vi "_fgv_rep_caps.vi"(5 "RepCapName in (\"\")":string, 6 "Repeated Capabilities (empty)":T1[](array[typedef]), 7 "Operation":T2=enum."Get Cmd Value", 8 "error in":errorcluster caption="error in (no error)", 9 "RepCapNameCmdValue in (\"\")":string, 10 "RepCapNameID in (\"\")":string, 11 "VISA resource name":refnum<visa-resource-name>) -> (0 "error out":errorcluster, 1 "RepCap count out":i32, 2 "CmdValue out":string, 3 "VISA resource name out":refnum<visa-resource-name>)   [LabVIEW 2020, in "Rohde&Schwarz RTx Oscilloscopes.lvlib" / "rsidr_core.lvlib"]
uses:
  rsidr_core.lvlib
  _type_Operation_Fgv_RepCap.ctl
  type_Input_Format_RepCap.ctl
  type_Error_Codes.ctl
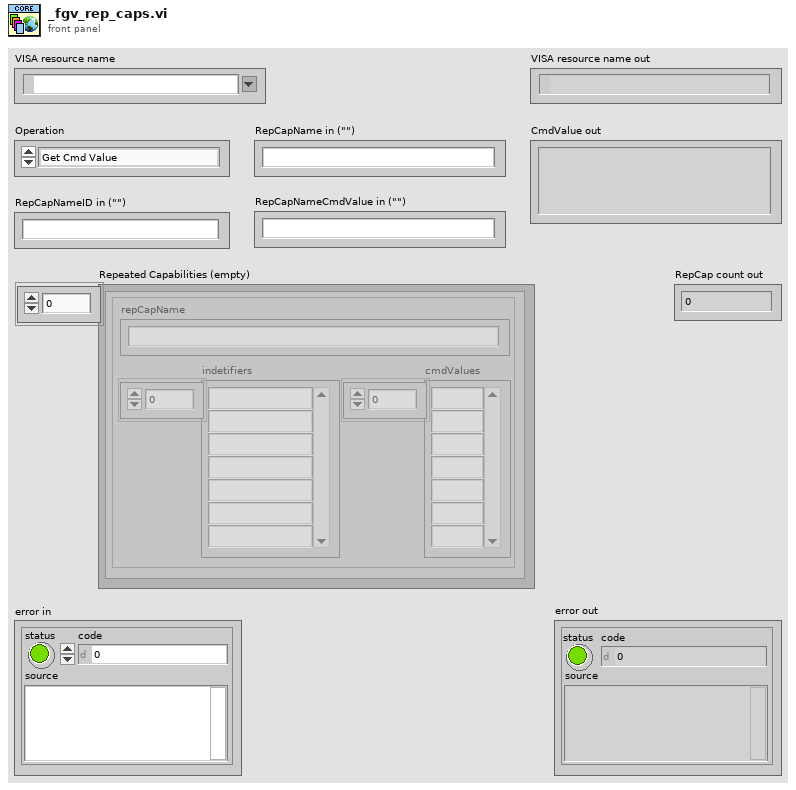
[diagram p1: front panel]
types:
  T1 = typedef "Rohde&Schwarz RTx Oscilloscopes.lvlib/rsidr_core.lvlib/type_Input_Format_RepCap.ctl" = cluster{"repCapName":string, "indetifiers":string[], "cmdValues":string[]}
  T2 = typedef "Rohde&Schwarz RTx Oscilloscopes.lvlib/rsidr_core.lvlib/_type_Operation_Fgv_RepCap.ctl" = enum16{"Initialize", "Get Cmd Value", "Reset Rep Cap", "Add Rep Cap", "Remove Rep Cap", "Get Rep Cap ID range", "Get Count", "Clear", "Find Name from NameID", "Get First NameID"}
  T3 = typedef "Rohde&Schwarz RTx Oscilloscopes.lvlib/rsidr_core.lvlib/type_Error_Codes.ctl" = enum16{"No_error", "VISA_err_ResourceNotFound", "VISA_err_Timeout", "VISA_warn_MoreDataAvailable", "RS_err_MissingCallback", "RS_err_InvalidAttribute", "RS_err_InvalidValue", "RS_err_UnknownResource", "RS_err_AlreadyInitialized", "RS_err_InstrumentStatus", "RS_err_BadRepCapName", "RS_err_TypesMismatch", "RS_err_ValueNotSupported", "RS_err_InvalidRngTable", "RS_err_IDqueryFail", "RS_err_UnexpResponse", "VISA_warn_ConfigNotLoaded", "RS_err_AttributeNotReadable", "RS_err_AttributeNotWritable", "RS_err_InstrumentType", "RS_err_InstrumentOption", "VISA_err_InvalidSize", "RS_err_ReliabilityIndicator", "VISA_warn_UnknownStatus", "VISA_warn_TermCharRead", "VISA_err_IO_error", "RS_err_FunctionNotSupported", "VISA_warn_QueueEmpty"}
  T4 = typedef "Rohde&Schwarz RTx Oscilloscopes.lvlib/rsidr_core.lvlib/_type_RepCap_Type.ctl" = enum16{"Arbitrary", "SequentialNull", "Sequential"}
  T5 = cluster{"repCapName":string, "RepCap Type out":T4, "RepCap IDs out":variant}
  T6 = cluster{"repCapName":string, "RepCap Type out":T4, "RepCap IDs out":variant}[]
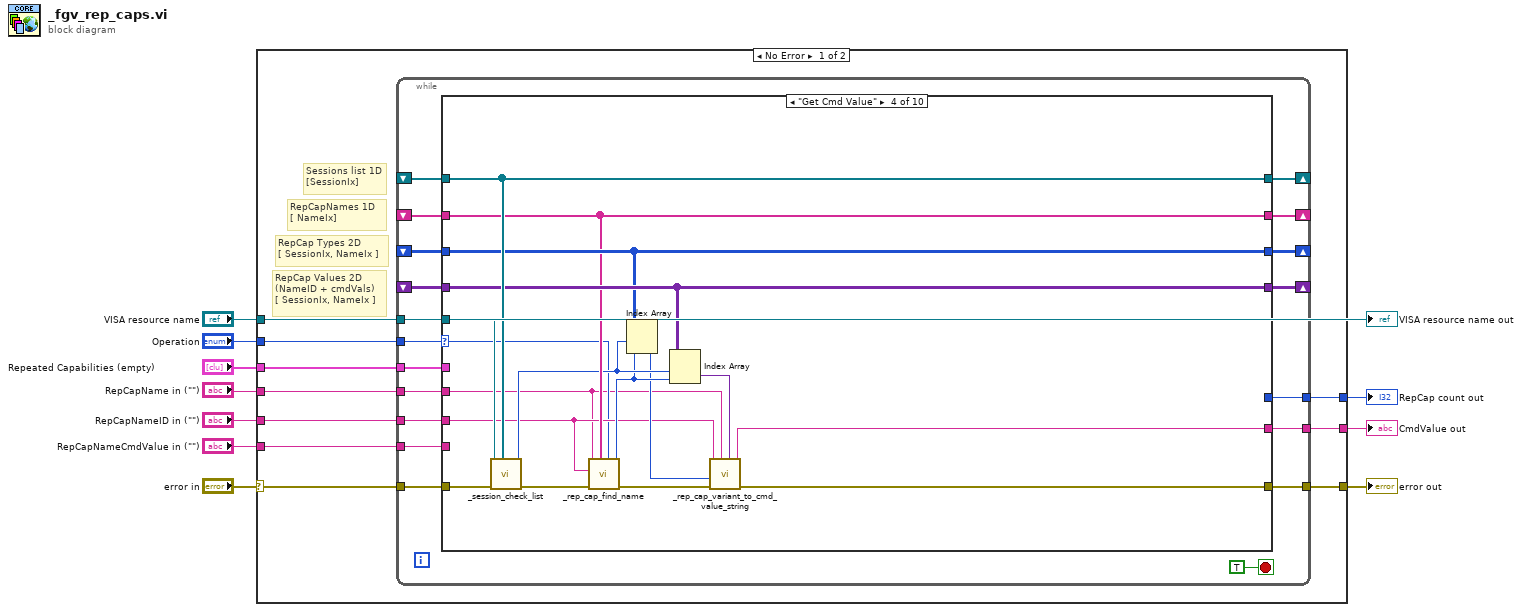
[diagram p0: block diagram]
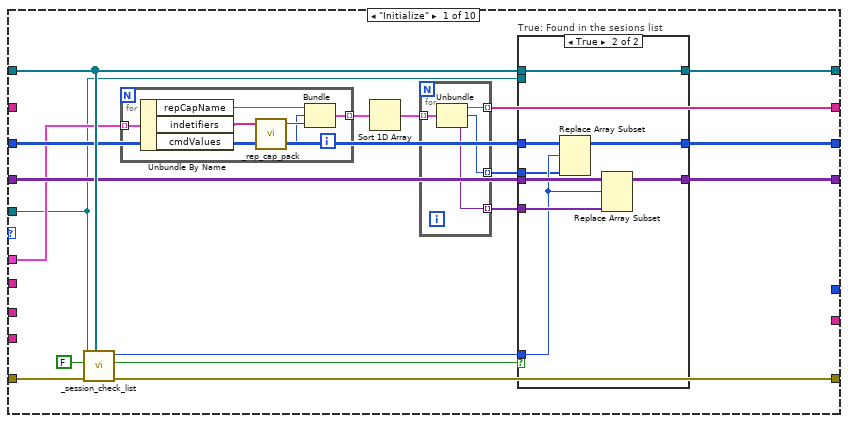
[diagram p2: hidden frame]
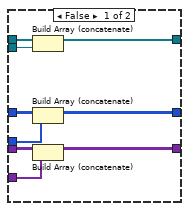
[diagram p3: hidden frame]
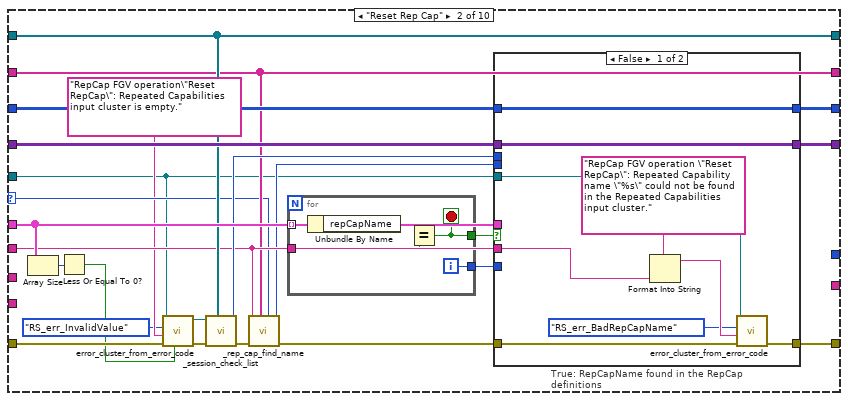
[diagram p4: hidden frame]
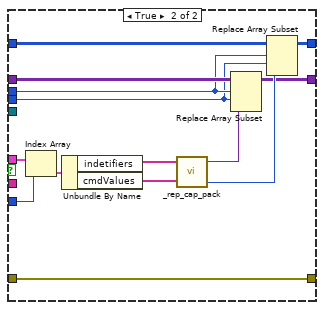
[diagram p5: hidden frame]
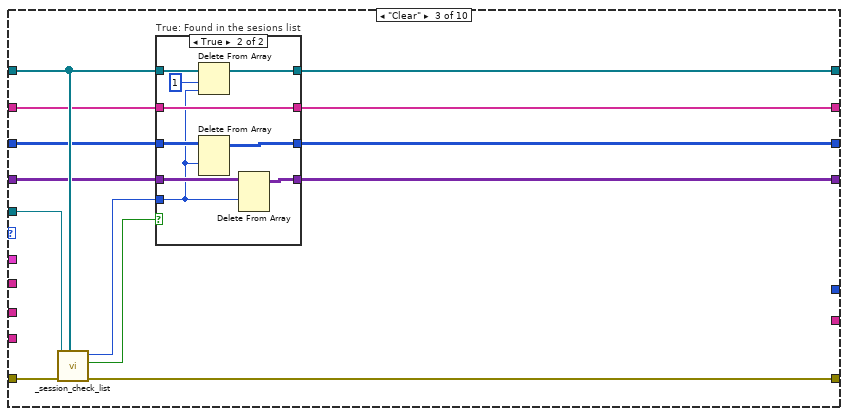
[diagram p6: hidden frame]
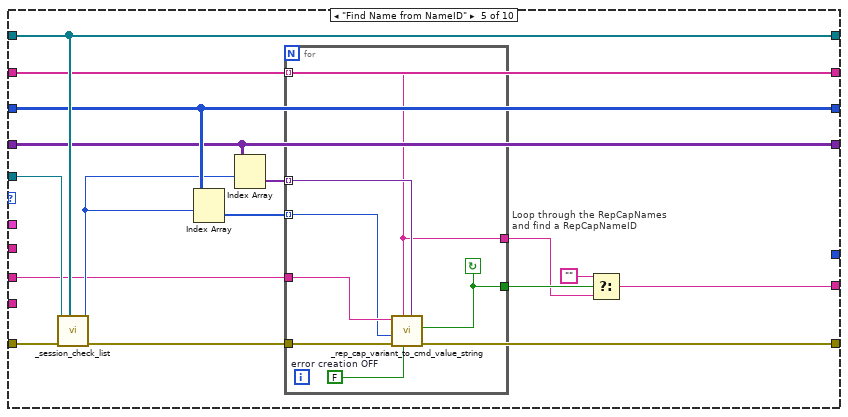
[diagram p8: hidden frame]
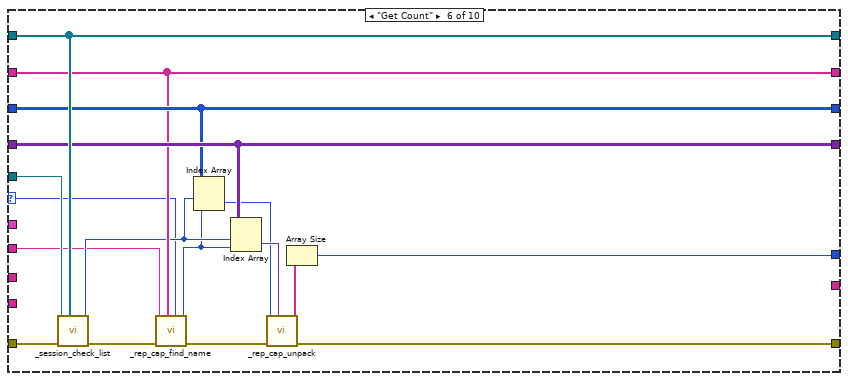
[diagram p9: hidden frame]
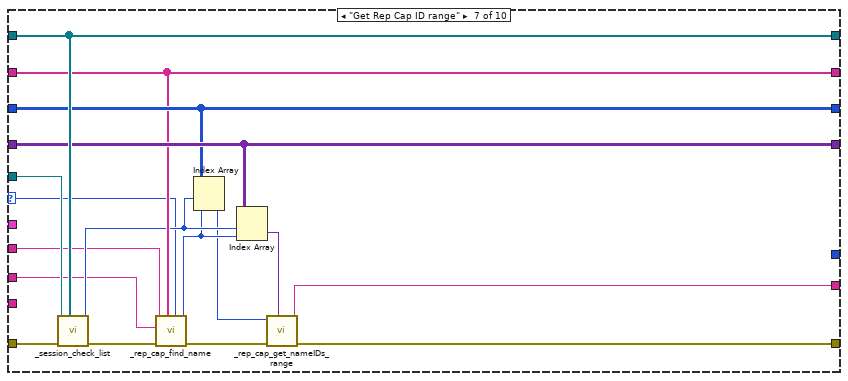
[diagram p10: hidden frame]
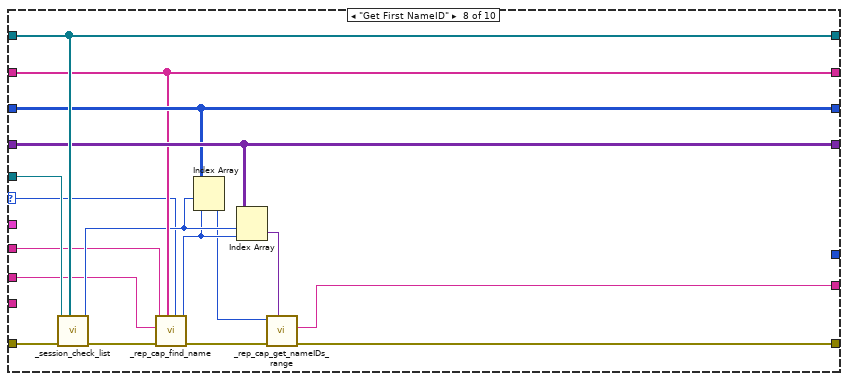
[diagram p11: hidden frame]
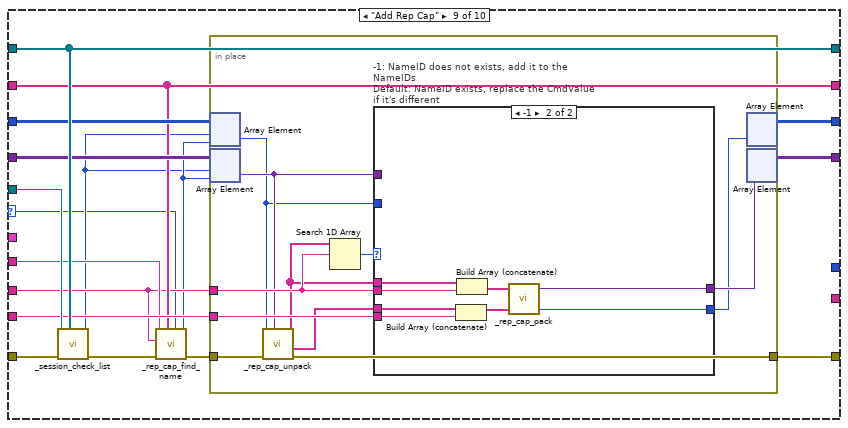
[diagram p12: hidden frame]
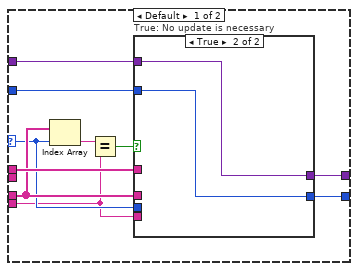
[diagram p13: hidden frame]
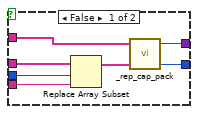
[diagram p14: hidden frame]
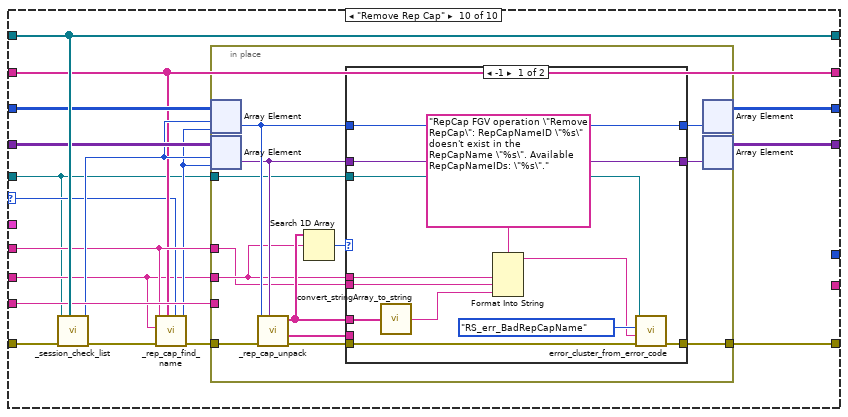
[diagram p15: hidden frame]
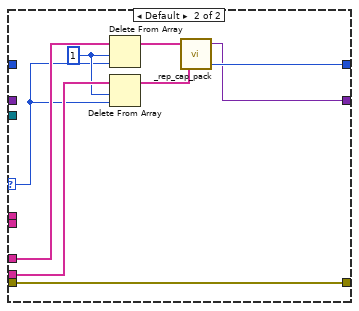
[diagram p16: hidden frame]
diagram:
  n1 = case shown="No Error" "error in" {
    selector: "error in" -> [w12 w360]
    tunnel: "Operation" -> [w20 _]
    tunnel: "VISA resource name" -> [w19 _]
    tunnel: [w13 w360] -> w9
    tunnel: "Repeated Capabilities (empty)" -> [w18 _]
    tunnel: "RepCapName in (\"\")" -> [w17 _]
    tunnel: "RepCapNameID in (\"\")" -> [w16 _]
    tunnel: [w15 _] -> w4
    tunnel: "RepCapNameCmdValue in (\"\")" -> [w14 _]
    tunnel: [w11 _] -> w1
    frame No Error {
      # "RepCap Values 2D\n(NameID + cmdVals)\n[ SessionIx, NameIx ]"
      # "Sessions list 1D\n[SessionIx]"
      # "RepCapNames 1D\n[ NameIx]"
      # "RepCap Types 2D\n[ SessionIx, NameIx ]"
      n2 = while {
        tunnel: w20 -> [w26]
        tunnel: [w39] -> w13
        tunnel: w19 -> [w23]
        tunnel: w18 -> [w37]
        tunnel: w17 -> [w36]
        tunnel: w16 -> [w35]
        tunnel: [w34] -> w15
        tunnel: w14 -> [w33]
        tunnel: w12 -> [w24]
        shift-right: [w31] -> _
        shift-left: _ -> [w32]
        shift-right: [w27] -> _
        shift-left: _ -> [w30]
        shift-right: [w28] -> _
        shift-left: _ -> [w29]
        shift-right: [w22] -> _
        shift-left: _ -> [w25]
        tunnel: [w21] -> w11
        stop <- TRUE stop-if-true
        n3 = case shown="\"Get Cmd Value\"" w26 {
          selector: w26 -> [_ w91 _ w165 _ w210 w227 w244 w254 w311]
          tunnel: [w56 w107 w149 w180 w185 w206 w222 w239 w270 w325] -> w39
          tunnel: w23 -> [w40 w86 w140 w177 w194 w218 w235 w252 w268 w309]
          tunnel: w37 -> [w43 w104 _ _ _ _ _ _ _ _]
          tunnel: w36 -> [_ w97 _ w164 _ w209 w226 w243 w259 w315]
          tunnel: w35 -> [_ _ _ w166 w187 _ w220 w238 w257 w310]
          tunnel: [_ _ _ w179 w182 _ w221 w237 _ _] -> w34
          tunnel: w33 -> [_ _ _ _ _ _ _ _ w262 w318]
          tunnel: w24 -> [w41 w109 w150 w178 w195 w219 w236 w253 w269 w324]
          tunnel: w32 -> [w48 w106 w141 w175 w190 w216 w233 w250 w266 w322]
          tunnel: [w45 w102 w138 w175 w190 w216 w233 w250 w263 w319] -> w31
          tunnel: w30 -> [_ w96 w145 w171 w191 w213 w230 w247 w258 w314]
          tunnel: w29 -> [w51 w105 w143 w174 w192 w215 w232 w249 w265 w321]
          tunnel: [w46 w103 w139 w174 w192 w215 w232 w249 w264 w320] -> w28
          tunnel: [w42 w96 w144 w171 w191 w213 w230 w247 w258 w314] -> w27
          tunnel: w25 -> [w53 w100 w147 w176 w193 w217 w234 w251 w267 w323]
          tunnel: [w52 w100 w146 w176 w193 w217 w234 w251 w267 w323] -> w22
          tunnel: [_ _ _ _ _ w204 _ _ _ _] -> w21
          frame "Initialize" {
            n4 = call "_session_check_list.vi"("VISA resource names in"=w53, "error in"=w41, "Error if not found (T)"=FALSE, "VISA resource name"=w40) -> ("error out"=w56:errorcluster, "Found in the list"=w54:bool, "Session list index out"=w50:i32)  [unwired: 5 in]
            n5 = for {
              tunnel: w43 -> [w85] mode=indexing
              tunnel: [w84] -> w55 mode=indexing
              n6 = Unbundle By Name(w85) -> ("repCapName"=w81:string, "indetifiers"=w83:string[], "cmdValues"=w79:string[])
              n7 = call "_rep_cap_pack.vi"("RepCapName CmdValues"=w79, "RepCapName IDs"=w83) -> ("RepCap Type out"=w80:T4, "RepCap IDs out"=w82:variant)  [unwired: 2 in]
              n8 = Bundle("repCapName"=w81, "RepCap Type out"=w80, "RepCap IDs out"=w82) -> (w84:T5)  [unwired: 1 in]
            }
            n9 = Sort 1D Array(array=w55) -> (sorted array=w57:T6)
            n10 = for {
              tunnel: w57 -> [w78] mode=indexing
              tunnel: [w76] -> w42 mode=indexing
              tunnel: [w77] -> w47 mode=indexing
              tunnel: [w75] -> w49 mode=indexing
              n11 = Unbundle(w78) -> ("repCapName"=w76:string, "RepCap Type out"=w77:T4, "RepCap IDs out"=w75:variant)
            }
            n12 = case "True: Found in the sesions list" shown="True" w54 {
              tunnel: w53 -> [w66 w74]
              tunnel: [w65 w74] -> w52
              tunnel: w51 -> [w63 w73]
              tunnel: w50 -> [_ w68]
              tunnel: w49 -> [w58 w71]
              tunnel: w48 -> [w61 w72]
              tunnel: w47 -> [w59 w67]
              tunnel: w40 -> [w64 _]
              tunnel: [w62 w70] -> w46
              tunnel: [w60 w69] -> w45
              frame False {
                n13 = Build Array (concatenate)(w66, w64) -> (w65:refnum<visa-resource-name>[])
                n14 = Build Array (concatenate)(w63, w59) -> (w62:T4[][])
                n15 = Build Array (concatenate)(w61, w58) -> (w60:variant[][])
              }
              frame True {
                n16 = Replace Array Subset(array=w73, new element=w67, index (row)=w68) -> (w70:T4[][])  [unwired: 1 in]
                n17 = Replace Array Subset(array=w72, new element=w71, index (row)=w68) -> (w69:variant[][])  [unwired: 1 in]
              }
            }
          }
          frame "Reset Rep Cap" {
            n18 = Array Size(array=w104) -> (size(s)=w108:i32)
            n19 = Less Or Equal To 0?(x=w108) -> (x <= 0?=w87:bool)
            n20 = call "error_cluster_from_error_code.vi"("Error Creation Enabled (True)"=w87, "error in"=w109, "Error Message (\"\")"="RepCap FGV operation\"Reset RepCap\": Repeated Capabilities input cluster is empty." ("format string"), "Error Enum in"=type_Error_Codes."RS_err_InvalidValue", "VISA resource name"=w86) -> ("error out"=w101:errorcluster, "VISA resource name out"=w90:refnum<visa-resource-name>)  [unwired: 5 in]
            n21 = call "_session_check_list.vi"("VISA resource names in"=w100, "error in"=w101, "VISA resource name"=w90) -> ("error out"=w98:errorcluster, "Session list index out"=w99:i32)  [unwired: 6 in, 1 out]
            n22 = call "_rep_cap_find_name.vi"("Operation for error msg"=w91, "RepCapNames in"=w96, "error in"=w98, "RepCapName to search"=w97) -> ("error out"=w94:errorcluster, "Index out"=w95:i32)  [unwired: 6 in]
            n23 = for {
              tunnel: w104 -> [w137] mode=indexing
              tunnel: w97 -> [w134]
              tunnel: [w133] -> w93
              tunnel: [w135] -> w92
              i -> [w135]
              stop <- w133 stop-if-true
              n24 = Unbundle By Name(w137) -> ("repCapName"=w136:string)
              n25 = Equal?(x=w136, y=w134) -> (x = y?=w133:bool)
            }
            n26 = case "True: RepCapName found in the RepCap definitions" shown="False" w93 {
              tunnel: w94 -> [w116 w119]
              tunnel: w104 -> [_ w131]
              tunnel: w92 -> [_ w132]
              tunnel: w105 -> [w118 w126]
              tunnel: w106 -> [w117 w123]
              tunnel: [w118 w127] -> w103
              tunnel: [w117 w124] -> w102
              tunnel: w99 -> [_ w122]
              tunnel: w95 -> [_ w121]
              tunnel: [w115 w119] -> w107
              tunnel: w97 -> [w113 _]
              tunnel: w86 -> [w112 _]
              frame False {
                n27 = Format Into String(format string="RepCap FGV operation \"Reset RepCap\": Repeated Capability name \"%s\" could not be found in the Repeated Capabilities input cluster.", w113) -> (resulting string=w111:string)  [unwired: 2 in, 1 out]
                n28 = call "error_cluster_from_error_code.vi"("error in"=w116, "Error Message (\"\")"=w111, "Error Enum in"=type_Error_Codes."RS_err_BadRepCapName", "VISA resource name"=w112) -> ("error out"=w115:errorcluster)  [unwired: 6 in, 1 out]
              }
              frame True {
                n29 = Index Array(array=w131, index=w132) -> (element=w130:T1)
                n30 = Unbundle By Name(w130) -> ("indetifiers"=w129:string[], "cmdValues"=w128:string[])
                n31 = call "_rep_cap_pack.vi"("RepCapName CmdValues"=w128, "RepCapName IDs"=w129) -> ("RepCap Type out"=w125:T4, "RepCap IDs out"=w120:variant)  [unwired: 2 in]
                n32 = Replace Array Subset(array=w123, new element=w120, index (row)=w122, index (col)=w121) -> (w124:variant[][])
                n33 = Replace Array Subset(array=w126, new element=w125, index (row)=w122, index (col)=w121) -> (w127:T4[][])
              }
            }
          }
          frame "Clear" {
            n34 = call "_session_check_list.vi"("VISA resource names in"=w147, "error in"=w150, "VISA resource name"=w140) -> ("error out"=w149:errorcluster, "Found in the list"=w148:bool, "Session list index out"=w142:i32)  [unwired: 6 in]
            n35 = case "True: Found in the sesions list" shown="True" w148 {
              tunnel: w147 -> [w154 w158]
              tunnel: [w154 w157] -> w146
              tunnel: w145 -> [w153 w159]
              tunnel: [w153 w159] -> w144
              tunnel: w143 -> [w152 w163]
              tunnel: w142 -> [_ w156]
              tunnel: w141 -> [w151 w162]
              tunnel: [w152 w161] -> w139
              tunnel: [w151 w160] -> w138
              frame False {
              }
              frame True {
                n36 = Delete From Array(array=w158, length=1, index=w156) -> (array with subset deleted=w157:refnum<visa-resource-name>[])  [unwired: 1 out]
                n37 = Delete From Array(array=w163, index (row)=w156) -> (array with subset deleted=w161:T4[][])  [unwired: 2 in, 1 out]
                n38 = Delete From Array(array=w162, index (row)=w156) -> (array with subset deleted=w160:variant[][])  [unwired: 2 in, 1 out]
              }
            }
          }
          frame "Get Cmd Value" {
            n39 = call "_session_check_list.vi"("VISA resource names in"=w176, "error in"=w178, "VISA resource name"=w177) -> ("error out"=w173:errorcluster, "Session list index out"=w170:i32)  [unwired: 6 in, 1 out]
            n40 = call "_rep_cap_find_name.vi"("Operation for error msg"=w165, "RepCapNames in"=w171, "error in"=w173, "RepCapNameID for error msg (\"\")"=w166, "RepCapName to search"=w164) -> ("error out"=w172:errorcluster, "Index out"=w169:i32)  [unwired: 5 in]
            n41 = Index Array(array=w174, index (row)=w170, index (col)=w169) -> (element=w168:T4)
            n42 = Index Array(array=w175, index (row)=w170, index (col)=w169) -> (element=w167:variant)
            n43 = call "_rep_cap_variant_to_cmd_value_string.vi"("RepCap value in"=w167, "RepCapName in"=w164, "error in"=w172, "RepCap Type in"=w168, "RepCapName ID in"=w166) -> ("error out"=w180:errorcluster, "CmdValue out"=w179:string)  [unwired: 4 in, 1 out]
          }
          frame "Find Name from NameID" {
            n44 = call "_session_check_list.vi"("VISA resource names in"=w193, "error in"=w195, "VISA resource name"=w194) -> ("error out"=w185:errorcluster, "Session list index out"=w189:i32)  [unwired: 6 in, 1 out]
            n45 = Index Array(array=w192, index (row)=w189) -> (element=w186:T4[])  [unwired: 1 in]
            n46 = Index Array(array=w190, index (row)=w189) -> (element=w188:variant[])  [unwired: 1 in]
            n47 = for "Loop through the RepCapNames\nand find a RepCapNameID" {
              tunnel: w191 -> [w198] mode=indexing
              tunnel: w188 -> [w201] mode=indexing
              tunnel: w187 -> [w202]
              tunnel: w186 -> [w200] mode=indexing
              tunnel: w185 -> [w199]
              tunnel: [w197] -> w184
              tunnel: [w198] -> w183
              stop <- w197 continue-if-true
              w196 = FALSE  # error creation OFF
              n48 = call "_rep_cap_variant_to_cmd_value_string.vi"("RepCap value in"=w201, "Error creation enabled (T)"=w196, "RepCapName in"=w198, "error in"=w199, "RepCap Type in"=w200, "RepCapName ID in"=w202) -> ("Error occured"=w197:bool)  [unwired: 3 in, 2 out]
            }
            n49 = Select(t="" ("Empty String Constant"), s=w184, f=w183) -> (s? t:f=w182:string)
          }
          frame "Get Count" {
            n50 = call "_session_check_list.vi"("VISA resource names in"=w217, "error in"=w219, "VISA resource name"=w218) -> ("error out"=w214:errorcluster, "Session list index out"=w212:i32)  [unwired: 6 in, 1 out]
            n51 = call "_rep_cap_find_name.vi"("Operation for error msg"=w210, "RepCapNames in"=w213, "error in"=w214, "RepCapName to search"=w209) -> ("error out"=w207:errorcluster, "Index out"=w211:i32)  [unwired: 6 in]
            n52 = Index Array(array=w215, index (row)=w212, index (col)=w211) -> (element=w203:T4)
            n53 = Index Array(array=w216, index (row)=w212, index (col)=w211) -> (element=w208:variant)
            n54 = call "_rep_cap_unpack.vi"("RepCap Value in"=w208, "error in"=w207, "RepCap Type in"=w203) -> ("error out"=w206:errorcluster, "RepCapName IDs"=w205:string[])  [unwired: 6 in, 1 out]
            n55 = Array Size(array=w205) -> (size(s)=w204:i32)
          }
          frame "Get Rep Cap ID range" {
            n56 = call "_session_check_list.vi"("VISA resource names in"=w234, "error in"=w236, "VISA resource name"=w235) -> ("error out"=w231:errorcluster, "Session list index out"=w229:i32)  [unwired: 6 in, 1 out]
            n57 = call "_rep_cap_find_name.vi"("Operation for error msg"=w227, "RepCapNames in"=w230, "error in"=w231, "RepCapNameID for error msg (\"\")"=w220, "RepCapName to search"=w226) -> ("error out"=w225:errorcluster, "Index out"=w228:i32)  [unwired: 5 in]
            n58 = Index Array(array=w232, index (row)=w229, index (col)=w228) -> (element=w224:T4)
            n59 = Index Array(array=w233, index (row)=w229, index (col)=w228) -> (element=w223:variant)
            n60 = call "_rep_cap_get_nameIDs_range.vi"("RepCap value in"=w223, "error in"=w225, "RepCap Type in"=w224) -> ("error out"=w222:errorcluster, "ID range out"=w221:string)  [unwired: 6 in, 1 out]
          }
          frame "Get First NameID" {
            n61 = call "_session_check_list.vi"("VISA resource names in"=w251, "error in"=w253, "VISA resource name"=w252) -> ("error out"=w248:errorcluster, "Session list index out"=w246:i32)  [unwired: 6 in, 1 out]
            n62 = call "_rep_cap_find_name.vi"("Operation for error msg"=w244, "RepCapNames in"=w247, "error in"=w248, "RepCapNameID for error msg (\"\")"=w238, "RepCapName to search"=w243) -> ("error out"=w242:errorcluster, "Index out"=w245:i32)  [unwired: 5 in]
            n63 = Index Array(array=w249, index (row)=w246, index (col)=w245) -> (element=w241:T4)
            n64 = Index Array(array=w250, index (row)=w246, index (col)=w245) -> (element=w240:variant)
            n65 = call "_rep_cap_get_nameIDs_range.vi"("RepCap value in"=w240, "error in"=w242, "RepCap Type in"=w241) -> ("error out"=w239:errorcluster, "First NameID out"=w237:string)  [unwired: 6 in, 1 out]
          }
          frame "Add Rep Cap" {
            n66 = call "_session_check_list.vi"("VISA resource names in"=w267, "error in"=w269, "VISA resource name"=w268) -> ("error out"=w261:errorcluster, "Session list index out"=w255:i32)  [unwired: 6 in, 1 out]
            n67 = call "_rep_cap_find_name.vi"("Operation for error msg"=w254, "RepCapNames in"=w258, "error in"=w261, "RepCapNameID for error msg (\"\")"=w257, "RepCapName to search"=w259) -> ("error out"=w260:errorcluster, "Index out"=w256:i32)  [unwired: 5 in]
            n68 = in-place "In Place Element Structure" {
              in-place-border: w260 -> [w281]
              in-place-border: w257 -> [w277]
              in-place-border: w262 -> [w280]
              in-place-border: [w278] -> w270
              n69 = in-place-array #1 ("Array Index / Replace Elements")(w265, w255, w256) -> (w272:T4)
              n70 = in-place-array #2 ("Array Index / Replace Elements")(w266, w255, w256) -> (w273:variant)
              n71 = call "_rep_cap_unpack.vi"("RepCap Value in"=w273, "error in"=w281, "RepCap Type in"=w272) -> ("error out"=w278:errorcluster, "RepCapCmdValues"=w279:string[], "RepCapName IDs"=w275:string[])  [unwired: 6 in]
              n72 = Search 1D Array(1D array=w275, element=w277) -> (index of element=w276:i32)  [unwired: 1 in]
              n73 = case "-1: NameID does not exists, add it to the NameIDs\nDefault: NameID exists, replace the CmdValue if it's different" shown="-1" w276 {
                selector: w276 -> [w283 _]
                tunnel: w280 -> [w282 w308]
                tunnel: w279 -> [w284 w307]
                tunnel: w277 -> [_ w306]
                tunnel: w275 -> [w287 w305]
                tunnel: [w290 w302] -> w274
                tunnel: [w289 w301] -> w271
                tunnel: w273 -> [w286 _]
                tunnel: w272 -> [w285 _]
                frame Default {
                  n74 = Index Array(array=w284, index=w283) -> (element=w291:string)
                  n75 = Equal?(x=w291, y=w282) -> (x = y?=w288:bool)
                  n76 = case "True: No update is necessary" shown="True" w288 {
                    tunnel: [w298 w300] -> w290
                    tunnel: [w297 w299] -> w289
                    tunnel: w287 -> [w296 _]
                    tunnel: w286 -> [_ w300]
                    tunnel: w285 -> [_ w299]
                    tunnel: w284 -> [w295 _]
                    tunnel: w283 -> [w294 _]
                    tunnel: w282 -> [w293 _]
                    frame False {
                      n77 = Replace Array Subset(array=w295, new element=w293, index=w294) -> (w292:string[])
                      n78 = call "_rep_cap_pack.vi"("RepCapName CmdValues"=w292, "RepCapName IDs"=w296) -> ("RepCap Type out"=w297:T4, "RepCap IDs out"=w298:variant)  [unwired: 2 in]
                    }
                    frame True {
                    }
                  }
                }
                frame -1 {
                  n79 = Build Array (concatenate)(w307, w308) -> (w303:string[])
                  n80 = Build Array (concatenate)(w305, w306) -> (w304:string[])
                  n81 = call "_rep_cap_pack.vi"("RepCapName CmdValues"=w303, "RepCapName IDs"=w304) -> ("RepCap Type out"=w301:T4, "RepCap IDs out"=w302:variant)  [unwired: 2 in]
                }
              }
              n82 = in-place-array #1 ("Array Index / Replace Elements")(w271) -> (w264:T4[][])  [unwired: 2 out]
              n83 = in-place-array #2 ("Array Index / Replace Elements")(w274) -> (w263:variant[][])  [unwired: 2 out]
            }
          }
          frame "Remove Rep Cap" {
            n84 = call "_session_check_list.vi"("VISA resource names in"=w323, "error in"=w324, "VISA resource name"=w309) -> ("error out"=w316:errorcluster, "Session list index out"=w317:i32)  [unwired: 6 in, 1 out]
            n85 = call "_rep_cap_find_name.vi"("Operation for error msg"=w311, "RepCapNames in"=w314, "error in"=w316, "RepCapNameID for error msg (\"\")"=w310, "RepCapName to search"=w315) -> ("error out"=w313:errorcluster, "Index out"=w312:i32)  [unwired: 5 in]
            n86 = in-place "In Place Element Structure" {
              in-place-border: w313 -> [w338]
              in-place-border: w310 -> [w331]
              in-place-border: w318 -> [_]
              in-place-border: [w334] -> w325
              in-place-border: w315 -> [w330]
              in-place-border: w309 -> [w326]
              n87 = in-place-array #3 ("Array Index / Replace Elements")(w321, w317, w312) -> (w337:T4)
              n88 = in-place-array #4 ("Array Index / Replace Elements")(w322, w317, w312) -> (w336:variant)
              n89 = call "_rep_cap_unpack.vi"("RepCap Value in"=w336, "error in"=w338, "RepCap Type in"=w337) -> ("error out"=w335:errorcluster, "RepCapCmdValues"=w327:string[], "RepCapName IDs"=w332:string[])  [unwired: 6 in]
              n90 = Search 1D Array(1D array=w332, element=w331) -> (index of element=w333:i32)  [unwired: 1 in]
              n91 = case shown="-1" w333 {
                selector: w333 -> [_ w351]
                tunnel: w337 -> [w345 _]
                tunnel: w336 -> [w344 _]
                tunnel: w335 -> [w350 w359]
                tunnel: [w349 w359] -> w334
                tunnel: w332 -> [w343 w356]
                tunnel: w331 -> [w347 _]
                tunnel: w330 -> [w346 _]
                tunnel: [w345 w358] -> w329
                tunnel: [w344 w357] -> w328
                tunnel: w327 -> [_ w354]
                tunnel: w326 -> [w340 _]
                frame -1 {
                  n92 = call "convert_stringArray_to_string.vi"("string array in"=w343) -> ("string out"=w339:string)  [unwired: 4 in]
                  n93 = Format Into String(format string="RepCap FGV operation \"Remove RepCap\": RepCapNameID \"%s\" doesn't exist in the RepCapName \"%s\". Available RepCapNameIDs: \"%s\".", w347, w346, w339) -> (resulting string=w341:string)  [unwired: 2 in, 1 out]
                  n94 = call "error_cluster_from_error_code.vi"("error in"=w350, "Error Message (\"\")"=w341, "Error Enum in"=type_Error_Codes."RS_err_BadRepCapName", "VISA resource name"=w340) -> ("error out"=w349:errorcluster)  [unwired: 6 in, 1 out]
                }
                frame Default {
                  w352 = 1 ("length")
                  n95 = Delete From Array(array=w356, length=w352, index=w351) -> (array with subset deleted=w355:string[])  [unwired: 1 out]
                  n96 = Delete From Array(array=w354, length=w352, index=w351) -> (array with subset deleted=w353:string[])  [unwired: 1 out]
                  n97 = call "_rep_cap_pack.vi"("RepCapName CmdValues"=w353, "RepCapName IDs"=w355) -> ("RepCap Type out"=w358:T4, "RepCap IDs out"=w357:variant)  [unwired: 2 in]
                }
              }
              n98 = in-place-array #3 ("Array Index / Replace Elements")(w329) -> (w320:T4[][])  [unwired: 2 out]
              n99 = in-place-array #4 ("Array Index / Replace Elements")(w328) -> (w319:variant[][])  [unwired: 2 out]
            }
          }
        }
      }
    }
    frame Error {
    }
  }
  "error out" <- w9
  "CmdValue out" <- w4
  "RepCap count out" <- w1
  "VISA resource name out" <- "VISA resource name"
